vi "Get name.vi"(8 "error in":errorcluster, 11 "Material-Scheme in":refnum<class "Material-Scheme.lvclass">) -> (0 "error out":errorcluster, 2 "name":string, 3 "Material-Scheme out":refnum<class "Material-Scheme.lvclass">)   [LabVIEW 2021, in "TSC Material Theme.lvlib" / "Material-Scheme.lvclass"]
doc: "Data member access method to read the name for the Scheme.\n\n<b>Code Developed By:</b>\nTechnology Service Corporation\n1983 S Liberty Drive\nBloomington, IN 47403\nwww.tsc.com/atcs\n\nDeveloper:\nDaniel Coons"
uses:
  Material-Scheme.lvclass
  Material-Scheme.lvclass/Material-Scheme.ctl
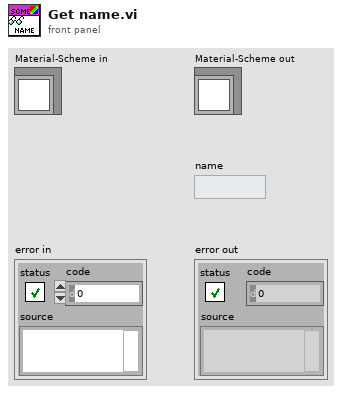
[diagram p1: front panel]
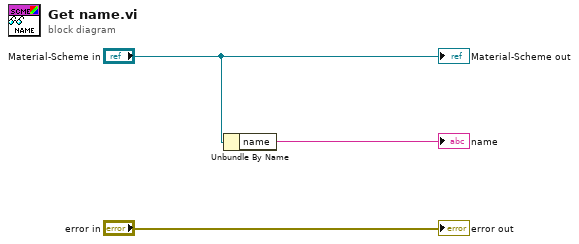
[diagram p0: block diagram]
diagram:
  n1 = Unbundle By Name("Material-Scheme in") -> ("name"=→"name":string)
  "error out" <- "error in"
  "Material-Scheme out" <- "Material-Scheme in"
